vi "Write Worktable.vi"(8 "error in":errorcluster, 10 "WorkTable":refnum<class "WorkTable Class.lvclass">, 11 "Gluing Procedure in":refnum<class "Gluing Procedure.lvclass">) -> (0 "error out":errorcluster, 3 "Gluing Procedure out":refnum<class "Gluing Procedure.lvclass">)   [LabVIEW 2011, in "Gluing Procedure.lvclass"]
uses:
  Gluing Procedure.lvclass
  Shared Components/WorkTable Class/WorkTable Class.lvclass
  Gluing Procedure.lvclass/Gluing Procedure.ctl
  Shared Components/Gantry Class/Gantry Class.lvclass
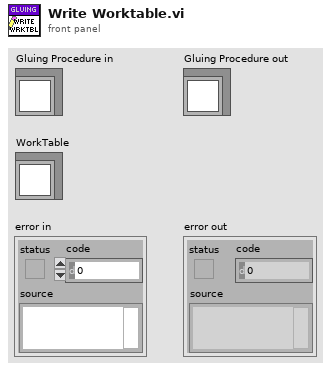
[diagram p1: front panel]
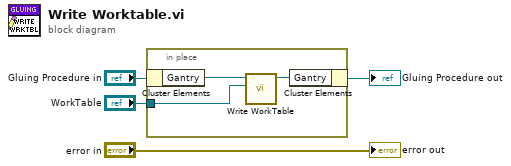
[diagram p0: block diagram]
diagram:
  n1 = in-place {
    in-place-border: "WorkTable" -> [w5]
    n2 = in-place-cluster #1("Gluing Procedure in") -> ("Gantry"=w6:refnum<class "Gantry Class.lvclass">)
    n3 = call-dynamic "Write WorkTable.vi"("WorkTable Class.lvclass"=w5, "Gantry Class in"=w6) -> ("Gantry Class out"=w7:refnum<class "Gantry Class.lvclass">)  [unwired: 8 in, 1 out]
    n4 = in-place-cluster #1("Gantry"=w7) -> (→"Gluing Procedure out":refnum<class "Gluing Procedure.lvclass">)
  }
  "error out" <- "error in"
